vi "Calculate possible moves.vi"(6 "Prune checked moves (T)":bool=TRUE, 7 "Position":refnum<class "Position.lvclass">, 8 "error in (no error)":errorcluster, 10 "Source":T1={"File"=enum."d", "Rank"=enum."4"}, 11 "Piece in":refnum<class "Piece.lvclass">) -> (0 "error out":errorcluster, 2 "Moves":refnum<class "Move.lvclass">[](array[class]), 3 "Piece out":refnum<class "Piece.lvclass">)   [LabVIEW 2016, in "Chesslib.lvlib" / "Piece.lvclass"]
uses:
  Piece.lvclass
  Position/Position.lvclass
  typedef/Square.ctl
  typedef/File.ctl
  typedef/Rank.ctl
  Moves/Move/Move.lvclass
  Chesslib.lvlib
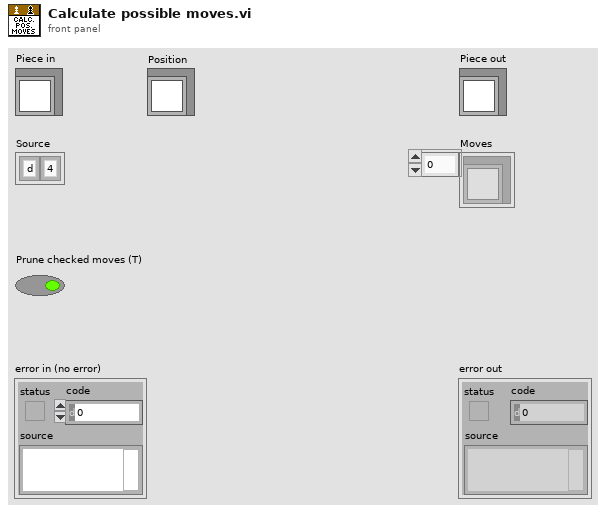
[diagram p1: front panel]
types:
  T1 = typedef "Chesslib.lvlib/Square.ctl" = cluster{"File":T2, "Rank":T3}
  T2 = typedef "Chesslib.lvlib/File.ctl" = enum8{"a", "b", "c", "d", "e", "f", "g", "h"}
  T3 = typedef "Chesslib.lvlib/Rank.ctl" = enum8{"1", "2", "3", "4", "5", "6", "7", "8"}
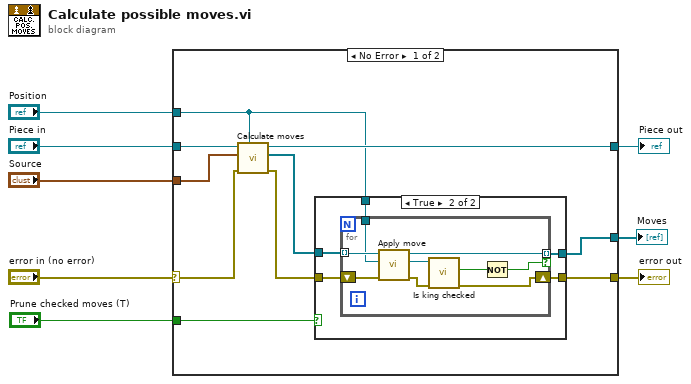
[diagram p0: block diagram]
diagram:
  n1 = case shown="No Error" "error in (no error)" {
    selector: "error in (no error)" -> [w15 w36]
    tunnel: [w10 w36] -> w7
    tunnel: [w17 w35] -> w5
    tunnel: "Piece in" -> [w18 w35]
    tunnel: "Position" -> [w13 _]
    tunnel: "Source" -> [w16 _]
    tunnel: [w12 _] -> w2
    tunnel: "Prune checked moves (T)" -> [w9 _]
    frame No Error {
      n2 = call-dynamic "Calculate moves.vi"("Position"=w13, "error in (no error)"=w15, "Source"=w16, "Piece in"=w18) -> ("error out"=w11:errorcluster, "Moves"=w14:refnum<class "Move.lvclass">[], "Piece out"=w17:refnum<class "Piece.lvclass">)  [unwired: 5 in]
      n3 = case shown="True" w9 {
        tunnel: w14 -> [w20 w25]
        tunnel: w13 -> [_ w24]
        tunnel: [w20 w23] -> w12
        tunnel: w11 -> [w19 w22]
        tunnel: [w19 w21] -> w10
        frame False {
        }
        frame True {
          n4 = for {
            tunnel: w25 -> [w34] mode=indexing
            tunnel: w24 -> [w33]
            tunnel: [w32] -> w23 mode=indexing if=w29
            shift-right: [w26] -> w21
            shift-left: w22 -> [w28]
            n5 = call "Apply move.vi"("error in (no error)"=w28, "Position in"=w33, "Move in"=w34) -> ("error out"=w27:errorcluster, "Position out"=w31:refnum<class "Position.lvclass">, "Move out"=w32:refnum<class "Move.lvclass">)  [unwired: 6 in]
            n6 = call "Is king checked.vi"("error in (no error)"=w27, "Position in"=w31) -> ("error out"=w26:errorcluster, "King is checked"=w30:bool)  [unwired: 7 in, 1 out]
            n7 = Not(x=w30) -> (.not. x?=w29:bool)
          }
        }
      }
    }
    frame Error {
    }
  }
  "error out" <- w7
  "Piece out" <- w5
  "Moves" <- w2
